vi "ConnectRobocad.vi"(8 "ErrorIn":errorcluster, 11 "Reference":T1) -> (0 "ErrorOut":errorcluster, 3 "OutConnection":T1)   [LabVIEW 2019]
uses:
  C:/Users/yasav/Downloads/prev_robocad/robocadSimLVFolder/assemblies/LibraryForLabVIEW.dll
  assemblies/LibraryForLabVIEW.dll
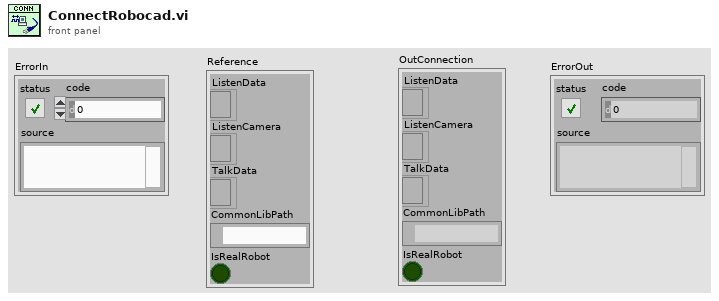
[diagram p1: front panel]
types:
  T1 = cluster{"ListenData":refnum<k24>, "ListenCamera":refnum<k24>, "TalkData":refnum<k24>, "CommonLibPath":path, "IsRealRobot":bool}
  T2 = cluster{"ListenData":refnum<k24>, "ListenCamera":refnum<k24>, "TalkData":refnum<k24>}
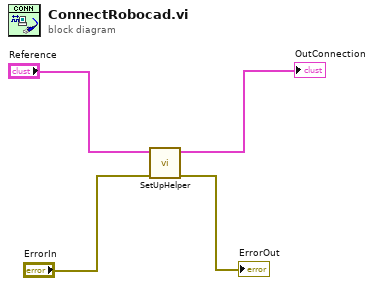
[diagram p0: block diagram]
diagram:
  n1 = call "SetUpHelper.vi"("ErrorIn"="ErrorIn", "Reference"="Reference") -> ("ErrorOut"=→"ErrorOut":errorcluster, "OutConnection"=→"OutConnection":T2)  [unwired: 8 in]
